vi "Green_Ana.vi"() -> ()   [LabVIEW 2011]
uses:
  <vilib>/DAQmx/write.llb/DAQmx Write (Analog DBL 1Chan 1Samp).vi
  <vilib>/DAQmx/create/channels.llb/DAQmx Create Channel (AO-Voltage-Basic).vi
  <vilib>/DAQmx/configure/timing.llb/DAQmx Timing (Sample Clock).vi
  <vilib>/DAQmx/miscellaneous.llb/DAQmx Fill In Error Info.vi
panel:
  in  "Green Laser Power":dbl
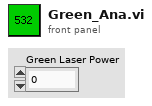
[diagram p1: front panel]
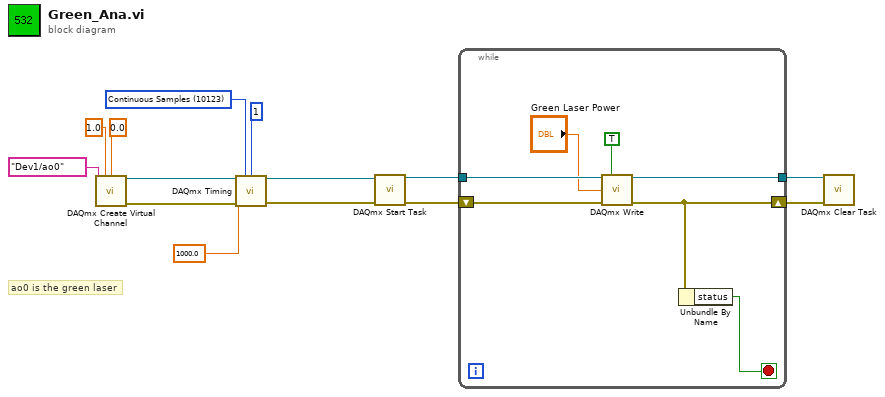
[diagram p0: block diagram]
diagram:
  w11 = 10123 items=["Finite Samples"=10178, "Continuous Samples"=10123, "Hardware Timed Single Point"=12522] ("sample mode")
  # "ao0 is the green laser"
  n1 = call-poly <vilib>:"DAQmx Create Virtual Channel.vi"("maximum value"=1.0, "minimum value"=0.0, "physical channels"=tag "Dev1/ao0") -> ("task out"=w8:refnum<k21>, "error out"=w7:errorcluster)  [unwired: 11 in]
  n2 = call-poly <vilib>:"DAQmx Timing.vi"("task/channels in"=w8, "sample mode"=w11, "samples per channel"=1, "rate"=1000.0, "error in"=w7) -> ("task out"=w6:refnum<k21>, "error out"=w5:errorcluster)  [unwired: 9 in]
  n3 = call <vilib>:"DAQmx Start Task.vi"("task/channels in"=w6, "error in"=w5) -> ("task out"=w4:refnum<k21>, "error out"=w1:errorcluster)  [unwired: 12 in]
  n4 = while {
    tunnel: w4 -> [w21]
    tunnel: [w17] -> w2
    shift-right: [w18] -> w3
    shift-left: w1 -> [w16]
    stop <- w19 stop-if-true
    n5 = call-poly <vilib>:"DAQmx Write.vi"("task/channels in"=w21, "auto start"=TRUE, "data"="Green Laser Power", "error in"=w16) -> ("task out"=w17:refnum<k21>, "error out"=w18:errorcluster)  [unwired: 9 in, 1 out]
    n6 = Unbundle By Name(w18) -> ("status"=w19:bool)
  }
  n7 = call <vilib>:"DAQmx Clear Task.vi"("task in"=w2, "error in"=w3) -> ()  [unwired: 13 in, 1 out]
